vi "NI 9237_Config.vi"(8 "error in":errorcluster, 11 "task in":refnum<k21>) -> (0 "error out":errorcluster, 3 "task out":refnum<k21>)   [LabVIEW 2022 SP3]
uses:
  <vilib>/DAQmx/create/channels.llb/DAQmx Create Channel (AI-Force-Bridge-Two-Point-Linear).vi
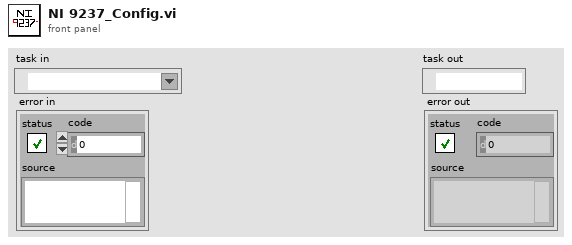
[diagram p1: front panel]
types:
  T1 = cluster{"bridge configuration":i32, "voltage excitation source":i32, "voltage excitation value":dbl, "nominal bridge resistance":dbl}
  T2 = cluster{"first electrical value":dbl, "second electrical value":dbl, "electrical units":i32, "first physical value":dbl, "second physical value":dbl, "physical units":i32}
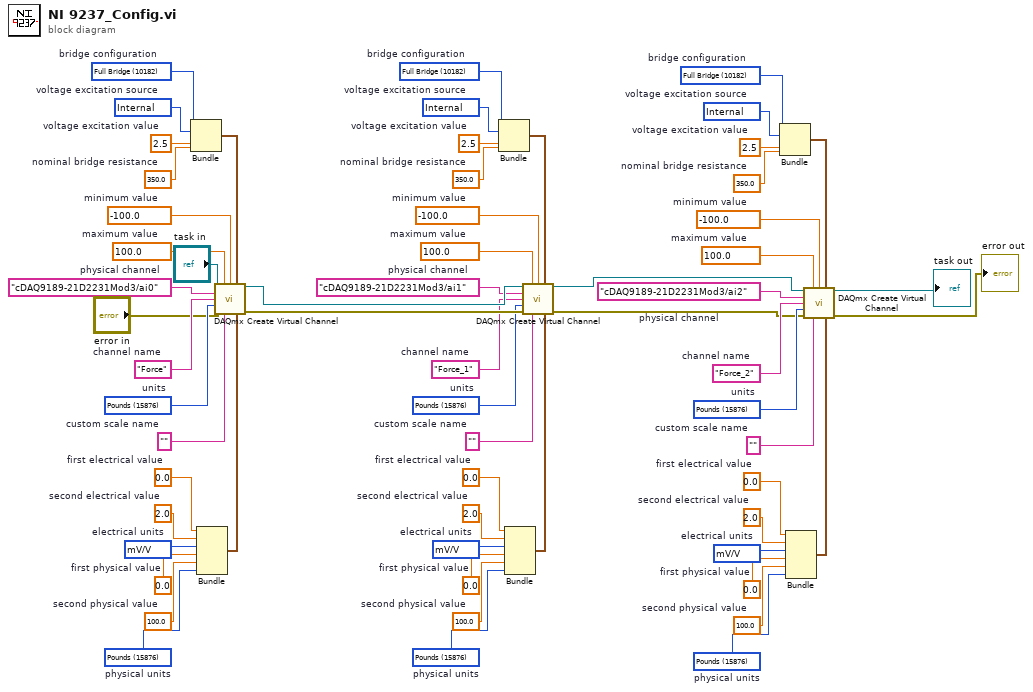
[diagram p0: block diagram]
diagram:
  w5 = 15876 items=["Newtons"=15875, "Pounds"=15876, "kgf"=15877]  # physical units
  w11 = 0.0  # first electrical value
  w10 = 2.0  # second electrical value
  w9 = 15897 items=["V/V"=15896, "mV/V"=15897]  # electrical units
  w8 = 0.0  # first physical value
  w7 = 100.0  # second physical value
  w13 = 350.0  # nominal bridge resistance
  w14 = 2.5  # voltage excitation value
  w15 = 10200 items=["Internal"=10200, "External"=10167]  # voltage excitation source
  w16 = 10182 items=["Full Bridge"=10182, "Half Bridge"=10187, "Quarter Bridge"=10270]  # bridge configuration
  w17 = 15876 items=["Newtons"=15875, "Pounds"=15876, "kgf"=15877, "From Custom Scale"=10065]  # units
  w18 = "Force_2"  # channel name
  w19 = ""  # custom scale name
  w20 = -100.0  # minimum value
  w21 = 100.0  # maximum value
  w22 = "cDAQ9189-21D2231Mod3/ai2"  # physical channel
  w25 = 15876 items=["Newtons"=15875, "Pounds"=15876, "kgf"=15877]  # physical units
  w31 = 0.0  # first electrical value
  w30 = 2.0  # second electrical value
  w29 = 15897 items=["V/V"=15896, "mV/V"=15897]  # electrical units
  w28 = 0.0  # first physical value
  w27 = 100.0  # second physical value
  w33 = 350.0  # nominal bridge resistance
  w34 = 2.5  # voltage excitation value
  w35 = 10200 items=["Internal"=10200, "External"=10167]  # voltage excitation source
  w36 = 10182 items=["Full Bridge"=10182, "Half Bridge"=10187, "Quarter Bridge"=10270]  # bridge configuration
  w37 = 15876 items=["Newtons"=15875, "Pounds"=15876, "kgf"=15877, "From Custom Scale"=10065]  # units
  w38 = "Force_1"  # channel name
  w39 = ""  # custom scale name
  w40 = -100.0  # minimum value
  w41 = 100.0  # maximum value
  w42 = "cDAQ9189-21D2231Mod3/ai1"  # physical channel
  w44 = 15876 items=["Newtons"=15875, "Pounds"=15876, "kgf"=15877]  # physical units
  w50 = 0.0  # first electrical value
  w49 = 2.0  # second electrical value
  w48 = 15897 items=["V/V"=15896, "mV/V"=15897]  # electrical units
  w47 = 0.0  # first physical value
  w46 = 100.0  # second physical value
  w52 = 350.0  # nominal bridge resistance
  w53 = 2.5  # voltage excitation value
  w54 = 10200 items=["Internal"=10200, "External"=10167]  # voltage excitation source
  w55 = 10182 items=["Full Bridge"=10182, "Half Bridge"=10187, "Quarter Bridge"=10270]  # bridge configuration
  w56 = 15876 items=["Newtons"=15875, "Pounds"=15876, "kgf"=15877, "From Custom Scale"=10065]  # units
  w57 = "Force"  # channel name
  w59 = ""  # custom scale name
  w60 = -100.0  # minimum value
  w61 = 100.0  # maximum value
  w62 = "cDAQ9189-21D2231Mod3/ai0"  # physical channel
  n1 = Bundle("bridge configuration"=w55, "voltage excitation source"=w54, "voltage excitation value"=w53, "nominal bridge resistance"=w52) -> (w51:T1)  [unwired: 1 in]
  n2 = Bundle("first electrical value"=w50, "second electrical value"=w49, "electrical units"=w48, "first physical value"=w47, "second physical value"=w46, "physical units"=w44) -> (w45:T2)  [unwired: 1 in]
  n3 = call-poly <vilib>:"DAQmx Create Virtual Channel.vi"("task in"="task in", "maximum value"=w61, "minimum value"=w60, "bridge information"=w51, "physical channels"=w62, "name to assign"=w57, "units"=w56, "error in"="error in", "custom scale name"=w59, "scaling information"=w45) -> ("task out"=w43:refnum<k21>, "error out"=w58:errorcluster)  [unwired: 4 in]
  n4 = Bundle("bridge configuration"=w36, "voltage excitation source"=w35, "voltage excitation value"=w34, "nominal bridge resistance"=w33) -> (w32:T1)  [unwired: 1 in]
  n5 = Bundle("first electrical value"=w31, "second electrical value"=w30, "electrical units"=w29, "first physical value"=w28, "second physical value"=w27, "physical units"=w25) -> (w26:T2)  [unwired: 1 in]
  n6 = call-poly <vilib>:"DAQmx Create Virtual Channel.vi"("task in"=w43, "maximum value"=w41, "minimum value"=w40, "bridge information"=w32, "physical channels"=w42, "name to assign"=w38, "units"=w37, "error in"=w58, "custom scale name"=w39, "scaling information"=w26) -> ("task out"=w4:refnum<k21>, "error out"=w3:errorcluster)  [unwired: 4 in]
  n7 = Bundle("bridge configuration"=w16, "voltage excitation source"=w15, "voltage excitation value"=w14, "nominal bridge resistance"=w13) -> (w12:T1)  [unwired: 1 in]
  n8 = Bundle("first electrical value"=w11, "second electrical value"=w10, "electrical units"=w9, "first physical value"=w8, "second physical value"=w7, "physical units"=w5) -> (w6:T2)  [unwired: 1 in]
  n9 = call-poly <vilib>:"DAQmx Create Virtual Channel.vi"("task in"=w4, "maximum value"=w21, "minimum value"=w20, "bridge information"=w12, "physical channels"=w22, "name to assign"=w18, "units"=w17, "error in"=w3, "custom scale name"=w19, "scaling information"=w6) -> ("task out"=→"task out":refnum<k21>, "error out"=→"error out":errorcluster)  [unwired: 4 in]
